vi "Result_Test.vi"(8 "error in (no error)":errorcluster caption="entrée d'erreur (pas d'erreur)", 11 "Flash_Jlink en entrée":refnum<class "Flash_Jlink.lvclass">) -> (0 "error out":errorcluster caption="sortie d'erreur", 3 "Flash_Jlink en sortie":refnum<class "Flash_Jlink.lvclass">)   [LabVIEW 2020, in "Library Test.lvlib" / "Flash_Jlink.lvclass"]
uses:
  Flash_Jlink.lvclass
  C:/Users/ngarcin/OneDrive - Altyor/Standard TB/Class/Test/Test (Default)/Test (Default).lvclass
  Test_Without_Instr/Test_Without_Inst.lvclass
  Flash_Jlink.lvclass/Flash_Jlink.ctl
panel:
  out "Allready Flash":bool
  out "standard output":string caption="sortie standard"
  out "Ok":bool
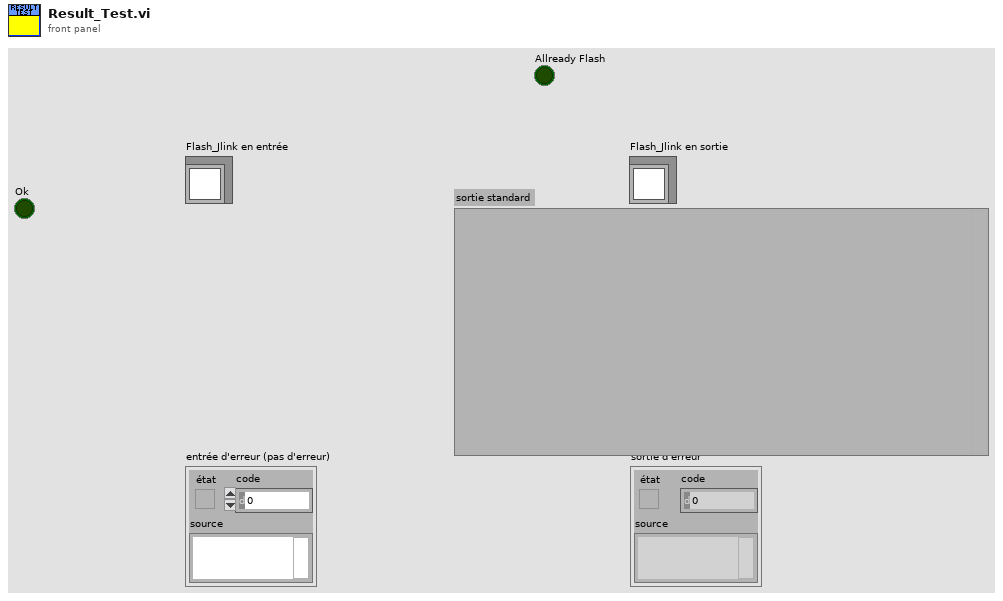
[diagram p1: front panel]
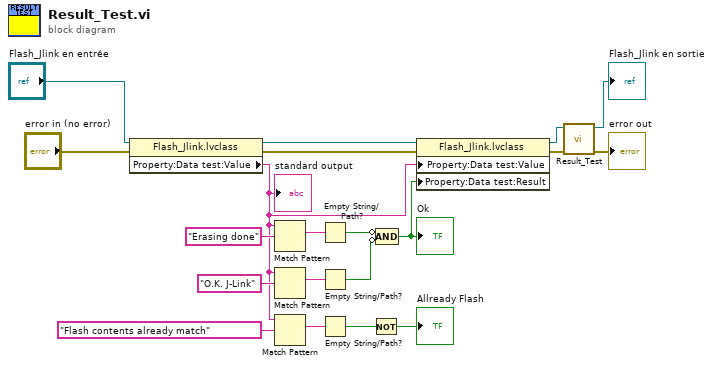
[diagram p0: block diagram]
diagram:
  n1 = property class="Flash_Jlink.lvclass"(reference="Flash_Jlink en entrée", error in="error in (no error)") -> (reference out=w4:refnum<class "Flash_Jlink.lvclass">, error out=w3:errorcluster, "Property:Data test:Value"=w9:string)
  "standard output" <- w9
  n2 = Match Pattern(string=w9, regular expression="Erasing done" ("expression régulière")) -> (match substring=w17:string)  [unwired: 1 in, 3 out]
  n3 = Match Pattern(string=w9, regular expression="O.K. J-Link" ("expression régulière")) -> (match substring=w19:string)  [unwired: 1 in, 3 out]
  n4 = Match Pattern(string=w9, regular expression="Flash contents already match" ("expression régulière")) -> (match substring=w13:string)  [unwired: 1 in, 3 out]
  n5 = Empty String/Path?(string/path=w17) -> (empty?=w15:bool)
  n6 = Empty String/Path?(string/path=w19) -> (empty?=w18:bool)
  n7 = Empty String/Path?(string/path=w13) -> (empty?=w12:bool)
  n8 = Not(x=w12) -> (.not. x?=→"Allready Flash":bool)
  n9 = Compound Arithmetic op=AND(invert w15, invert w18) -> (w10:bool)
  "Ok" <- w10
  n10 = property class="Flash_Jlink.lvclass"(reference=w4, error in=w3, "Property:Data test:Value"=w9, "Property:Data test:Result"=w10) -> (reference out=w2:refnum<class "Flash_Jlink.lvclass">, error out=w6:errorcluster)
  n11 = call-parent "Result_Test.vi"("error in (no error)"=w6, "Test_Without_Inst en entrée"=w2) -> ("error out"=→"error out":errorcluster, "Test_Without_Inst en sortie"=→"Flash_Jlink en sortie":refnum<class "Flash_Jlink.lvclass">)  [unwired: 8 in]
